vi "ObstacleEnemyRadius.vi"(4 "Goal":dbl[](array[numeric]), 6 "Initial State":dbl[](array[numeric]), 9 "Robot enemy":T1={"id"=0, "function"=enum."Attacker", "x"=0.0, "y"=0.0, "orientation"=0.0, "v_tangent"=0.0, "v_normal"=0.0, "v_ang"=0.0, "kick_x"=0.0, "kick_z"=0.0, "dribble"=FALSE, "Timestamp"=timestamp(0 s since 1904-01-01), "estimatives"={"est_v_tangent"=0.0, "est_v_normal"=0.0, "est_vx"=0.0, "est_vy"=0.0, "Pos Robot Est"=[]}, "dest_x_kick"=0.0, "dest_y_kick"=0.0, "Gap Coord"=[], "States"=enum."GoToTangent", "Path "=[], "Path  Smooth"=[], "Dest"=[], "vx_desired"=0.0, "vy_desired"=0.0, "slowBehavior"=FALSE, "VSSStates"=enum."Pass"}, 10 "Robot in":T1={"id"=0, "function"=enum."Attacker", "x"=0.0, "y"=0.0, "orientation"=0.0, "v_tangent"=0.0, "v_normal"=0.0, "v_ang"=0.0, "kick_x"=0.0, "kick_z"=0.0, "dribble"=FALSE, "Timestamp"=timestamp(0 s since 1904-01-01), "estimatives"={"est_v_tangent"=0.0, "est_v_normal"=0.0, "est_vx"=0.0, "est_vy"=0.0, "Pos Robot Est"=[]}, "dest_x_kick"=0.0, "dest_y_kick"=0.0, "Gap Coord"=[], "States"=enum."GoToTangent", "Path "=[], "Path  Smooth"=[], "Dest"=[], "vx_desired"=0.0, "vy_desired"=0.0, "slowBehavior"=FALSE, "VSSStates"=enum."Pass"}) -> (2 "obstacle enemy radius":dbl)   [LabVIEW 2023]
uses:
  Vision_class/Old vision/Controls/AI Robot.ctl
  Vision_class/Old vision/Controls/Functions Enum.ctl
  Vision_class/Old vision/Controls/AttackerStates.ctl
  Vision_class/Old vision/Controls/PathDests.ctl
  Vision_class/Old vision/Controls/PathDest.ctl
  Navigation/VSSNavigation/VSSAttackerStates.ctl
  <vilib>/Analysis/_algsub.llb/Real Vector Norm.vi
  <vilib>/Analysis/NI_AALPro.lvlib
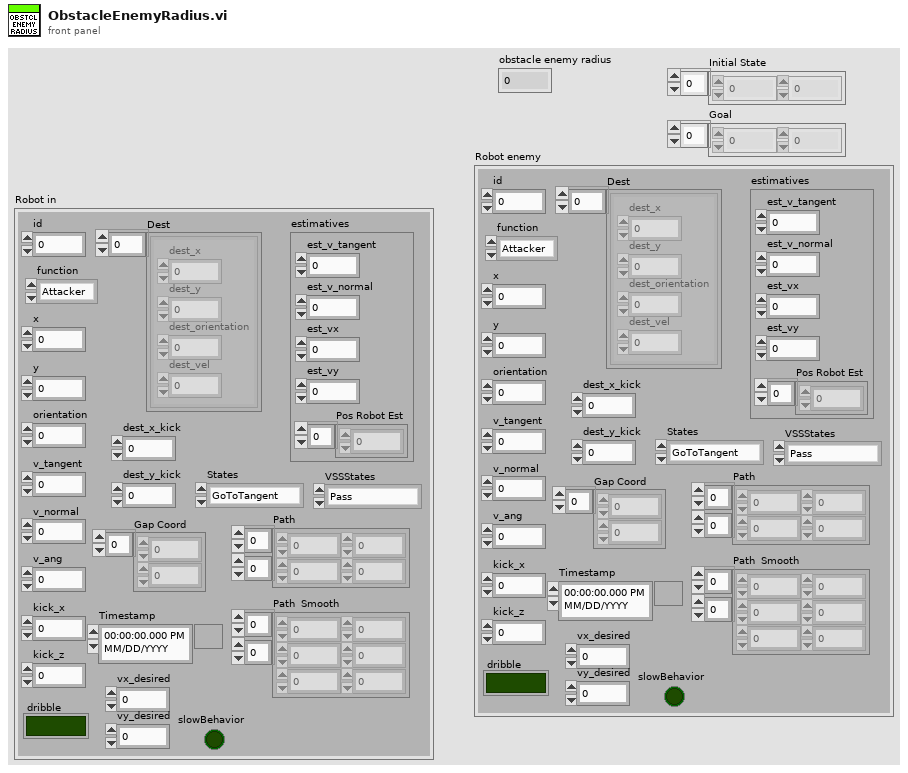
[diagram p1: front panel]
types:
  T1 = typedef "AI Robot.ctl" = cluster{"id":u32, "function":T2, "x":dbl, "y":dbl, "orientation":dbl, "v_tangent":dbl, "v_normal":dbl, "v_ang":dbl, "kick_x":dbl, "kick_z":dbl, "dribble":bool, "Timestamp":timestamp, "estimatives":cluster{"est_v_tangent":dbl, "est_v_normal":dbl, "est_vx":dbl, "est_vy":dbl, "Pos Robot Est":dbl[]}, "dest_x_kick":dbl, "dest_y_kick":dbl, "Gap Coord":dbl[], "States":T3, "Path ":dbl[][], "Path  Smooth":dbl[][], "Dest":T4, "vx_desired":dbl, "vy_desired":dbl, "slowBehavior":bool, "VSSStates":T6}
  T2 = typedef "Functions Enum.ctl" = enum16{"2nd Striker", "Attacker", "Goalie", "Defender", "Striker", "Goto 0", "Dummy", "Kicker", "ZigZag 0", "ZigZag 1", "ZigZag 2", "ZigZag 3", "ZigZag 4", "ZigZag 5", "ZigZag 6", "ZigZag 7", "ZigZag 8", ""}
  T3 = typedef "AttackerStates.ctl" = enum16{"Pass", "GoToTangent", "BallGetting", "GoToKick", ""}
  T4 = typedef "PathDests.ctl" = T5[]
  T5 = typedef "PathDest.ctl" = cluster{"dest_x":dbl, "dest_y":dbl, "dest_orientation":dbl, "dest_vel":dbl}
  T6 = typedef "VSSAttackerStates.ctl" = enum16{"Pass", "GoToTangent", "BallGetting", "GoToKick", "Rotate anti-clockwise", "Rotate Clockwise", ""}
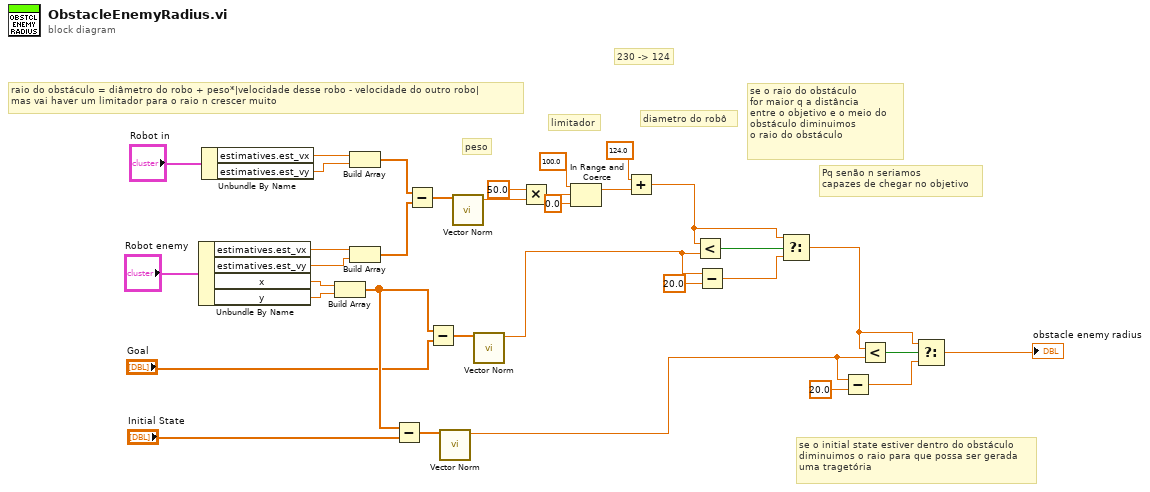
[diagram p0: block diagram]
diagram:
  # "230 -> 124"
  # "se o initial state estiver dentro do obstáculo\ndiminuimos o raio para que possa ser gerada\numa tragetória"
  # "limitador"
  # "peso"
  # "diametro do robô"
  # "Pq senão n seriamos\ncapazes de chegar no objetivo"
  # "se o raio do obstáculo\nfor maior q a distância \nentre o objetivo e o meio do \nobstáculo diminuimos \no raio do obstáculo"
  # "raio do obstáculo = diâmetro do robo + peso*|velocidade desse robo - velocidade do outro robo|\nmas vai haver um limitador para o raio n crescer muito"
  n1 = Unbundle By Name("Robot enemy") -> ("estimatives.est_vx"=w32:dbl, "estimatives.est_vy"=w31:dbl, "x"=w18:dbl, "y"=w17:dbl)
  n2 = Unbundle By Name("Robot in") -> ("estimatives.est_vx"=w30:dbl, "estimatives.est_vy"=w29:dbl)
  n3 = Build Array(w18, w17) -> (w9:dbl[])
  n4 = Build Array(w30, w29) -> (w28:dbl[])
  n5 = Build Array(w32, w31) -> (w27:dbl[])
  n6 = Subtract(x=w9, y="Initial State") -> (x-y=w10:dbl[])
  n7 = Subtract(x=w28, y=w27) -> (x-y=w26:dbl[])
  n8 = Subtract(x=w9, y="Goal") -> (x-y=w16:dbl[])
  n9 = call-poly <vilib>:"Vector Norm.vi"("Input Vector"=w10) -> ("norm"=w3:dbl)  [unwired: 9 in, 1 out]
  n10 = call-poly <vilib>:"Vector Norm.vi"("Input Vector"=w26) -> ("norm"=w25:dbl)  [unwired: 9 in, 1 out]
  n11 = call-poly <vilib>:"Vector Norm.vi"("Input Vector"=w16) -> ("norm"=w13:dbl)  [unwired: 9 in, 1 out]
  n12 = Multiply(x=50.0, y=w25) -> (x*y=w23:dbl)
  n13 = In Range and Coerce(upper limit=100.0, x=w23, lower limit=0.0) -> (coerced(x)=w20:dbl)  [unwired: 1 out]
  n14 = Add(x=124.0, y=w20) -> (x+y=w14:dbl)
  n15 = Less?(x=w14, y=w13) -> (x < y?=w15:bool)
  n16 = Subtract(x=w13, y=20.0) -> (x-y=w11:dbl)
  n17 = Select(t=w14, s=w15, f=w11) -> (s? t:f=w5:dbl)
  n18 = Subtract(x=w3, y=20.0) -> (x-y=w2:dbl)
  n19 = Less?(x=w5, y=w3) -> (x < y?=w7:bool)
  n20 = Select(t=w5, s=w7, f=w2) -> (s? t:f=→"obstacle enemy radius":dbl)
